vi "DAC_setAllOutputs.vi"(8 "error in (no error)":errorcluster, 9 "outputs":u32[](array[numeric]), 10 "isIr":bool, 11 "drvno":u32) -> (0 "error out":errorcluster)   [LabVIEW 2015, in "ESLSCDLL.lvlib"]
uses:
  ESLSCDLL.lvlib
  ESLSCDLL.dll
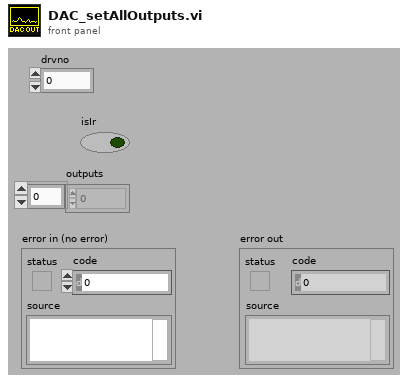
[diagram p1: front panel]
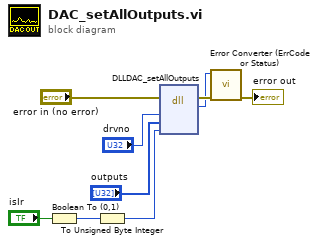
[diagram p0: block diagram]
diagram:
  n1 = Boolean To (0,1)(Boolean="isIr") -> (0, 1=w4:i16)
  n2 = To Unsigned Byte Integer(number=w4) -> (unsigned 8bit integer=w2:u8)
  n3 = dll-call lib="C:/ENTW/PCIE/LV64/board.vis/ESLSCDLL.dll" fn="DLLDAC_setAllOutputs" ("lwlscdll.dll:DLLSetADAmpRed")(error in="error in (no error)", "drvno"="drvno", "outputs"="outputs", "isIr"=w2) -> (error out=w7:errorcluster, "es_status_codes"=w6:i32)  [unwired: 5 in, 1 out]
  n4 = call "Error Converter (ErrCode or Status).vi"("error in (no error)"=w7, "error code"=w6) -> ("error out"=→"error out":errorcluster)  [unwired: 9 in]
